vi "数据查询.vi"() -> ()   [LabVIEW 2016]
uses:
  <vilib>/Utility/miscctls.llb/LVPointTypeDef.ctl
panel:
  in  "数据查询菜单":enum32{"数据查询", "仪器数据", "仪器日志", "报警信息", "校准查询"}(xcontrol)
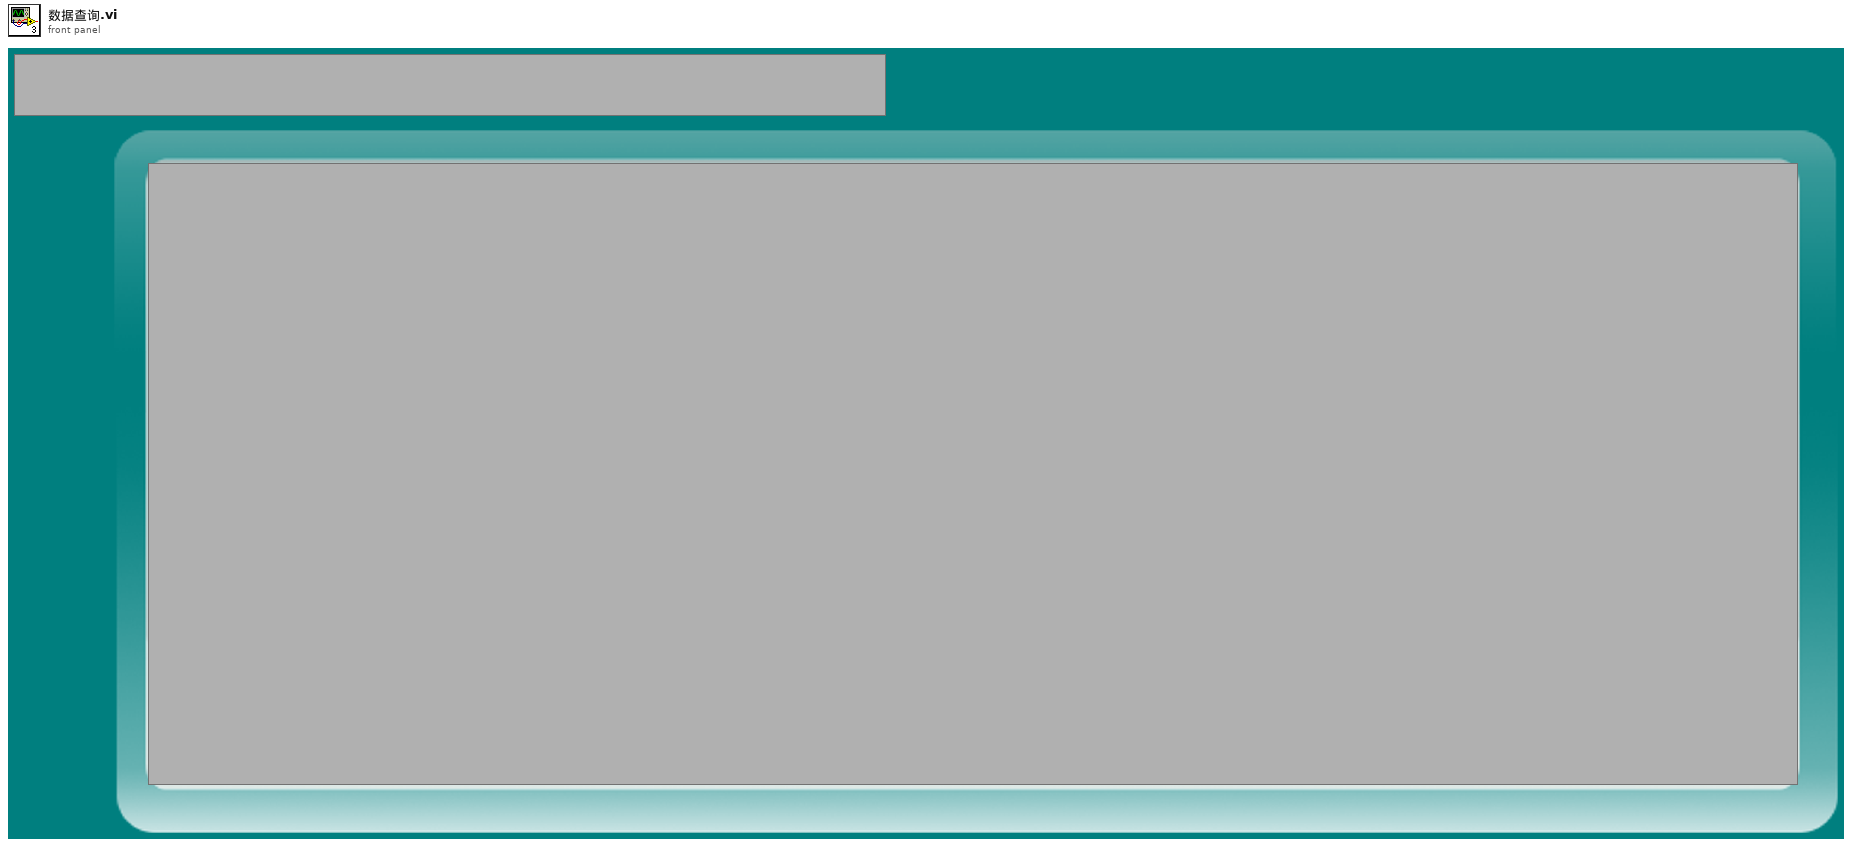
[diagram p1: front panel]
types:
  T1 = typedef "LVPointTypeDef.ctl" = cluster{"Horizontal":i16, "Vertical":i16}
  T2 = enum32{"Bad", "Idle", "Run top level", "Running"}
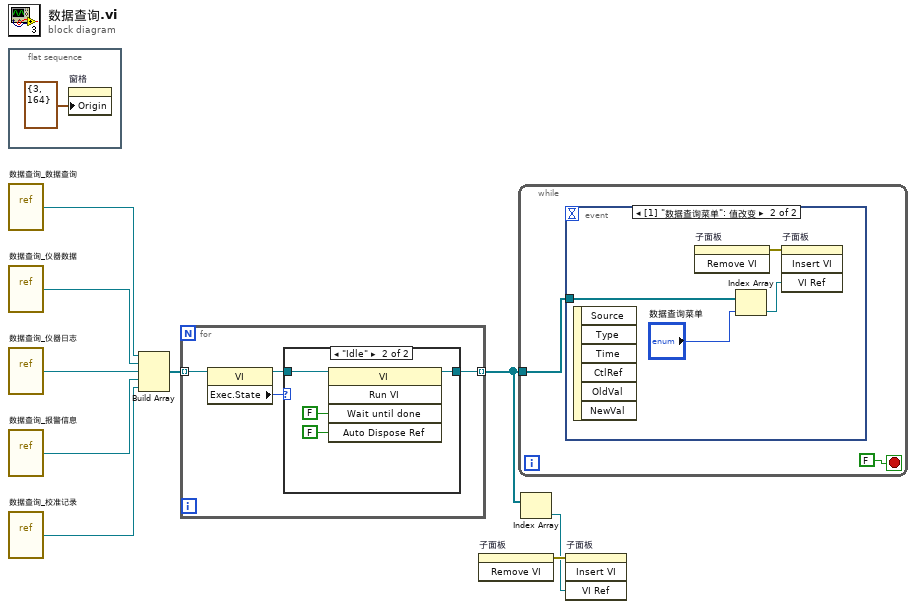
[diagram p0: block diagram]
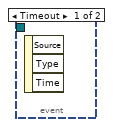
[diagram p3: hidden frame]
diagram:
  n1 = flat-sequence {
    frame #0 {
      n2 = property on="窗格" class="Pane"("Origin"=T1 {"Horizontal"=3, "Vertical"=164} ("原点")) -> ()  [unwired: 2 in, 2 out]
    }
  }
  n3 = vi-ref "数据查询_数据查询.vi"() -> (w6:refnum<vi>)
  n4 = vi-ref "数据查询_仪器数据.vi"() -> (w4:refnum<vi>)
  n5 = vi-ref "数据查询_仪器日志.vi"() -> (w3:refnum<vi>)
  n6 = vi-ref "数据查询_报警信息.vi"() -> (w2:refnum<vi>)
  n7 = vi-ref "数据查询_校准记录.vi"() -> (w1:refnum<vi>)
  n8 = Build Array(w6, w4, w3, w2, w1) -> (w5:refnum<vi>[])
  n9 = for {
    tunnel: w5 -> [w14] mode=indexing
    tunnel: [w11] -> w8 mode=indexing
    n10 = property class="VI"(reference=w14) -> (reference out=w12:refnum<vi>, "Exec.State"=w13:T2)  [unwired: 1 in, 1 out]
    n11 = case shown="\"Idle\"" w13 {
      tunnel: w12 -> [w15 w17]
      tunnel: [w15 w16] -> w11
      frame "Bad", Default {
      }
      frame "Idle" {
        n12 = invoke class="VI" method="Run VI"(reference=w17, "Wait until done"=FALSE ("结束前等待"), "Auto Dispose Ref"=FALSE ("自动销毁引用")) -> (reference out=w16:refnum<vi>)  [unwired: 2 in, 4 out]
      }
    }
  }
  n13 = invoke on="子面板" class="SubPnl" method="Remove VI"() -> (error out=w9:errorcluster)  [unwired: 3 in, 2 out]
  n14 = while {
    tunnel: w8 -> [w20]
    stop <- FALSE stop-if-true
    n15 = event shown="[1] \"数据查询菜单\": 值改变" {
      selector: _ -> [_ _]
      dyn-events: _ -> [_ _]
      timeout: _ -> [_ _]
      tunnel: w20 -> [_ w25]
      event Timeout {
        n16 = event-data() -> ()  [unwired: 1 in, 3 out]
      }
      event "数据查询菜单": Value Change {
        n17 = event-data() -> ()  [unwired: 1 in, 6 out]
        n18 = invoke on="子面板" class="SubPnl" method="Remove VI"() -> (error out=w22:errorcluster)  [unwired: 3 in, 2 out]
        n19 = Index Array(array=w25, index="数据查询菜单") -> (element=w23:refnum<vi>)
        n20 = invoke on="子面板" class="SubPnl" method="Insert VI"(error in=w22, "VI Ref"=w23) -> ()  [unwired: 2 in, 4 out]
      }
    }
  }
  n21 = Index Array(array=w8) -> (element=w7:refnum<vi>)  [unwired: 1 in]
  n22 = invoke on="子面板" class="SubPnl" method="Insert VI"(error in=w9, "VI Ref"=w7) -> ()  [unwired: 2 in, 4 out]
